vi "NI 5114 Example_aab.vi"() -> ()   [LabVIEW 2018]
uses:
  <instrlib>/niScope/Acquire/Fetch/niScope Multi Fetch Cluster.vi
  <instrlib>/niScope/Configure/Trigger/niScope Configure Trigger Window.vi
  <instrlib>/niScope/Acquire/Fetch/niScope Fetch.vi
panel:
  in  "STOP":bool
  out "SEU_Counter":u32 caption="SEU counter"
  out "SEU":bool caption="SEL"
  out "SEU Waveform":T1(graph) caption="SHUTDOWN Waveform"
  out "SEU Last Level":dbl
  out "RealTime Waveform":T1(graph) caption="PC_MON Waveform"
  in  "Low Level":dbl=0.35 format="%.2f"
  in  "High Level":dbl=0.65 format="%.2f"
  in  "Trigger Source":string(combo)="0"
  in  "AC/DC/Ground":i32(ring)=1 items=["AC", "DC", "Ground"]
  in  "vertical range":dbl=2.0 caption="Vertical Range" format="%.2f"
  out "NI Scope error out":errorcluster
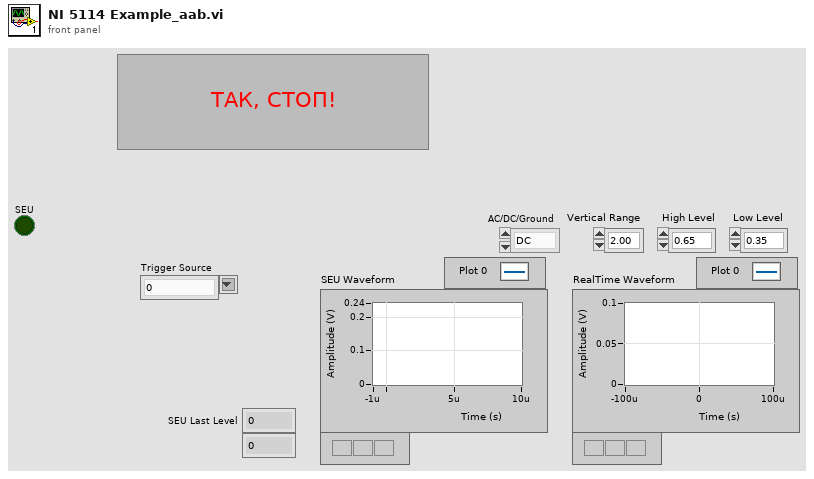
[diagram p1: front panel]
types:
  T1 = cluster{"relativeInitialX":dbl, "xIncrement":dbl, "wfm":dbl[]}[]
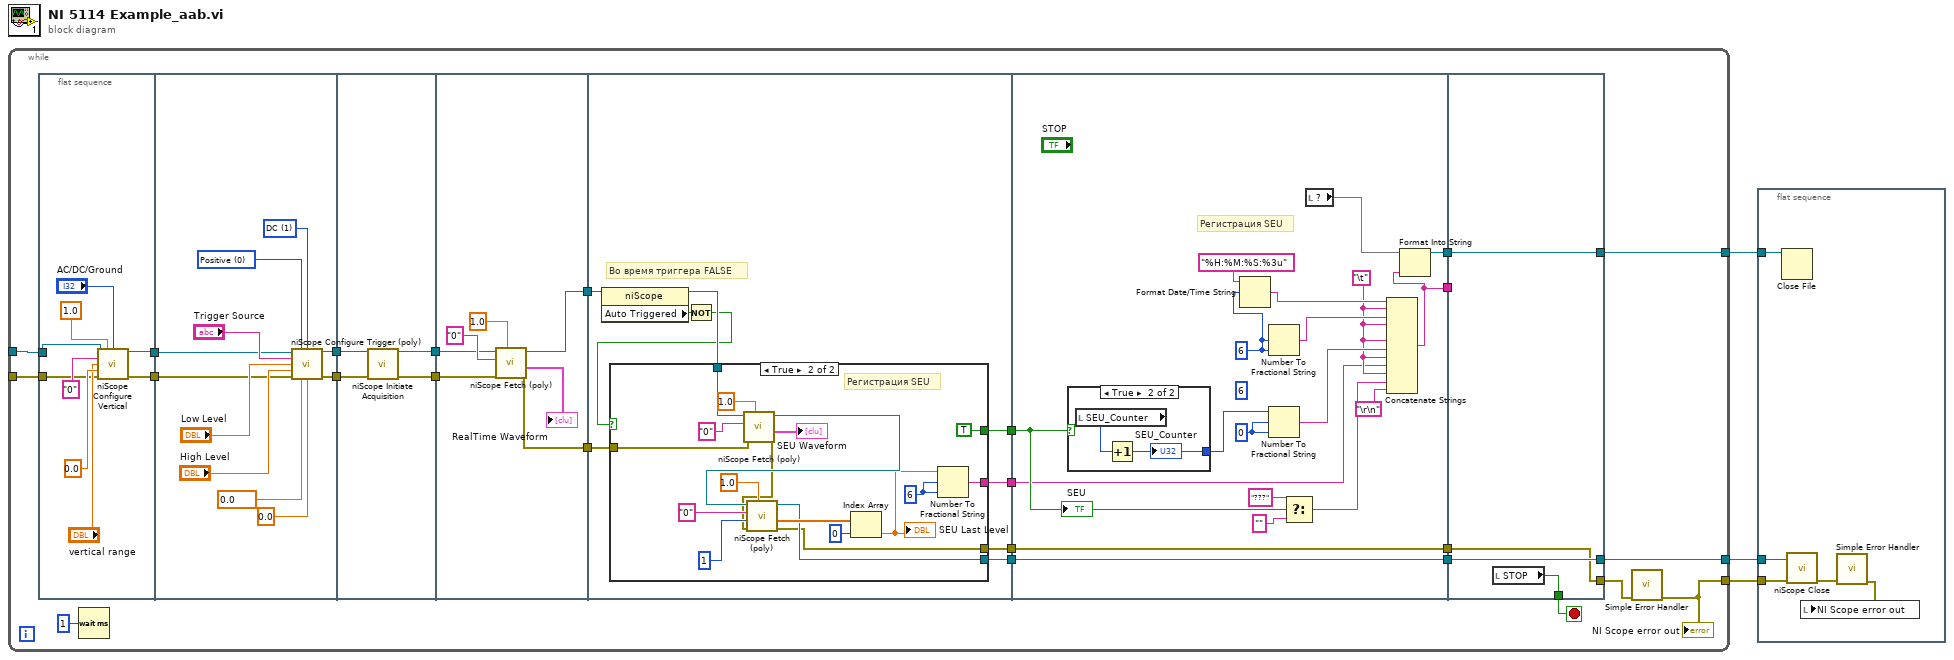
[diagram p0: block diagram]
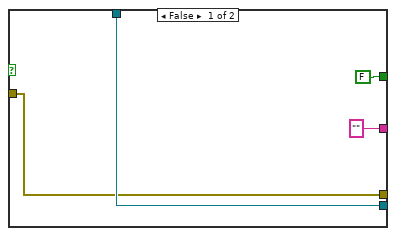
[diagram p2: hidden frame]
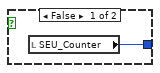
[diagram p3: hidden frame]
diagram:
  n1 = while {
    tunnel: _ -> [w22]
    tunnel: [w27] -> w2
    tunnel: [w16] -> w1
    tunnel: [w4] -> w3
    tunnel: _ -> [w6]
    stop <- w23 stop-if-true
    n2 = flat-sequence {
      tunnel: w22 -> [w35]
      tunnel: [w32] -> w14
      tunnel: w6 -> [w29]
      tunnel: [w28] -> w12
      tunnel: [w42] -> w26
      tunnel: w14 -> [w41]
      tunnel: w12 -> [w38]
      tunnel: [w37] -> w11
      tunnel: [w51] -> w25
      tunnel: w26 -> [w50]
      tunnel: w11 -> [w49]
      tunnel: [w48] -> w10
      tunnel: w25 -> [w55]
      tunnel: [w54] -> w24
      tunnel: w10 -> [w53]
      tunnel: [w52] -> w9
      tunnel: [w65] -> w20
      tunnel: w24 -> [w67]
      tunnel: [w64] -> w18
      tunnel: [w62] -> w13
      tunnel: w9 -> [w61]
      tunnel: [w60] -> w7
      tunnel: w20 -> [w109]
      tunnel: [w109] -> w19
      tunnel: w18 -> [w97]
      tunnel: [w101] -> w17
      tunnel: [w99] -> w15
      tunnel: w13 -> [w95]
      tunnel: [w92] -> w8
      tunnel: w7 -> [w92]
      tunnel: [w115] -> w27
      tunnel: w19 -> [w115]
      tunnel: [w116] -> w23
      tunnel: w17 -> [w114]
      tunnel: [w114] -> w16
      tunnel: w15 -> [_]
      tunnel: w8 -> [w113]
      tunnel: [w113] -> w5
      frame #0 {
        n3 = call <instrlib>:"niScope Configure Vertical.vi"("instrument handle"=w35, "probe attenuation"=1.0 ("Probe Attenuation"), "vertical coupling"="AC/DC/Ground", "channels"="0" ("Channel Name"), "vertical range"="vertical range", "vertical offset"=0.0, "error in"=w29) -> ("instrument handle out"=w32:refnum<k15>, "error out"=w28:errorcluster)  [unwired: 7 in]
      }
      frame #1 {
        w47 = 0 items=["Positive", "Negative"] ("Trigger Slope")
        w46 = u16 1 items=["AC"=0, "DC"=1, "HF Reject"=3, "LF Reject"=4, "AC Plus HF Reject"=1001] ("Coupling")
        n4 = call-poly <instrlib>:"niScope Configure Trigger (poly).vi"("instrument handle"=w41, "trigger window mode"=w47, "trigger coupling"=w46, "trigger source"="Trigger Source", "low level"="Low Level", "high level"="High Level", "error in"=w38, "trigger holdoff"=0.0, "trigger delay"=0.0 ("Trigger Delay")) -> ("instrument handle out"=w42:refnum<k15>, "error out"=w37:errorcluster)  [unwired: 5 in]
      }
      frame #2 {
        n5 = call <instrlib>:"niScope Initiate Acquisition.vi"("instrument handle"=w50, "error in"=w49) -> ("instrument handle out"=w51:refnum<k15>, "error out"=w48:errorcluster)  [unwired: 12 in]
      }
      frame #3 {
        n6 = call-poly <instrlib>:"niScope Fetch (poly).vi"("timeout"=1.0, "error in"=w53, "channels"="0", "instrument handle"=w55) -> ("error out"=w52:errorcluster, "waveform"=→"RealTime Waveform":T1, "instrument handle out"=w54:refnum<k15>)  [unwired: 4 in, 1 out]
      }
      frame #4 {
        # "Во время триггера FALSE"
        n7 = property class="niScope"(reference=w67) -> (reference out=w66:refnum<k15>, "Auto Triggered"=w63:bool)  [unwired: 1 in, 1 out]
        n8 = Not(x=w63) -> (.not. x?=w59:bool)
        n9 = case shown="True" w59 {
          tunnel: w66 -> [w71 w86]
          tunnel: [w71 w78] -> w65
          tunnel: [FALSE TRUE] -> w64
          tunnel: ["" w75] -> w62
          tunnel: w61 -> [w68 w74]
          tunnel: [w68 w72] -> w60
          frame False {
          }
          frame True {
            w77 = 6
            # "Регистрация SEU"
            n10 = call-poly <instrlib>:"niScope Fetch (poly).vi"("timeout"=1.0, "error in"=w74, "channels"="0", "instrument handle"=w86) -> ("error out"=w73:errorcluster, "waveform"=→"SEU Waveform":T1, "instrument handle out"=w79:refnum<k15>)  [unwired: 4 in, 1 out]
            n11 = call-poly <instrlib>:"niScope Fetch (poly).vi"("timeout"=1.0, "error in"=w73, "numSamples"=1, "channels"="0", "instrument handle"=w79) -> ("error out"=w72:errorcluster, "wfm"=w84:dbl[], "instrument handle out"=w78:refnum<k15>)  [unwired: 3 in, 1 out]
            n12 = Index Array(array=w84, index=0) -> (element=w76:dbl)
            "SEU Last Level" <- w76
            n13 = Number To Fractional String(number=w76, width (-)=w77, precision (6)=w77) -> (F-format string=w75:string)  [unwired: 1 in]
          }
        }
      }
      frame #5 {
        w90 = 6
        w104 = 0
        (unwired) 6
        w96 = "\t"
        # "Регистрация SEU"
        n14 = case shown="True" w97 {
          tunnel: [w110 w111] -> w98
          frame False {
            n15 = local read "SEU_Counter"() -> (w110:u32)
          }
          frame True {
            n16 = local read "SEU_Counter"() -> (w112:u32)
            n17 = Increment(x=w112) -> (x+1=w111:u32)
            "SEU_Counter" <- w111
          }
        }
        n18 = Format Date/Time String(time format string (%c)="%H:%M:%S:%3u", seconds (now)=w90) -> (date/time string=w106:string)  [unwired: 1 in]
        n19 = Number To Fractional String(width (-)=w90, precision (6)=w90) -> (F-format string=w105:string)  [unwired: 2 in]
        n20 = Number To Fractional String(number=w98, width (-)=w104, precision (6)=w104) -> (F-format string=w108:string)  [unwired: 1 in]
        n21 = Select(t="???", s=w97, f="") -> (s? t:f=w94:string)
        n22 = local read item#-1() -> (w91)
        n23 = Concatenate Strings(w106, w96, w105, w96, w96, w108, w96, w95, w96, w94, "\r\n") -> (w99:string, w107:string)
        n24 = Format Into String(initial string=w91, w99) -> (resulting string=w101:refnum<file>)  [unwired: 2 in, 1 out]
        "SEU" <- w97
      }
      frame #6 {
        n25 = local read "STOP"() -> (w116:bool)
      }
    }
    n26 = Wait (ms)(milliseconds to wait=u32 1) -> ()  [unwired: 1 out]
    n27 = call <vilib>:"Simple Error Handler.vi"("error in (no error)"=w5) -> ("error out"=w4:errorcluster)  [unwired: 1 in, 7 out]
    "NI Scope error out" <- w4
  }
  n28 = flat-sequence {
    tunnel: w2 -> [w121]
    tunnel: [w117] -> _
    tunnel: w3 -> [w120]
    tunnel: w1 -> [w117]
    frame #0 {
      n29 = Close File(refnum=w117) -> ()  [unwired: 1 in, 2 out]
      n30 = call <instrlib>:"niScope Close.vi"("instrument handle"=w121, "error in"=w120) -> ("error out"=w119:errorcluster)  [unwired: 13 in]
      n31 = call <vilib>:"Simple Error Handler.vi"("error in (no error)"=w119) -> ("error out"=w118:errorcluster)  [unwired: 1 in, 7 out]
      n32 = local write "NI Scope error out"(w118) -> ()
    }
  }
